vi "Field_C process Set field cmd.vi"(7 "Magnet Constants":T8, 10 "PSU Status in":T1 {"Trip Current" format="%.3f"; "Trip Field" format="%.4f"; "Voltage" format="%.2f"; "Field Constant" format="%.6f"; "MID Setpoint (T)" format="%.4f"; "MID Setpoint (A)" format="%.3f"; "MAX Setpoint (T)" format="%.4f"; "MAX Setpoint (A)" format="%.3f"; "Heater Voltage" format="%.2f"; "V Limit (V)" format="%.2f"; "Ramp Rate (A/s)" format="%.3f"; "Output (A)" format="%.3f"; "Output (T)" format="%.4f"; "Persistent Current" format="%.3f"; "Persistent Field" format="%.4f"}, 11 "Overall status in":T4) -> (2 "PSU Status Out out":T1 {"Trip Current" format="%.3f"; "Trip Field" format="%.4f"; "Voltage" format="%.2f"; "Field Constant" format="%.6f"; "MID Setpoint (T)" format="%.4f"; "MID Setpoint (A)" format="%.3f"; "MAX Setpoint (T)" format="%.4f"; "MAX Setpoint (A)" format="%.3f"; "Heater Voltage" format="%.2f"; "V Limit (V)" format="%.2f"; "Ramp Rate (A/s)" format="%.3f"; "Output (A)" format="%.3f"; "Output (T)" format="%.4f"; "Persistent Current" format="%.3f"; "Persistent Field" format="%.4f"}, 3 "Overall status out":T4)   [LabVIEW 2024, in "Magnet module.lvlib"]
uses:
  Magnet module.lvlib
  ctl/Magnet mode public.ctl
  ctl/SetField data.ctl
  ctl/Magnet config constants.ctl
  ctl/Magnet mode.ctl
  ctl/RampingOutput.ctl
  ctl/Actual magnet state.ctl
  ctl/Overall status.ctl
  <instrlib>/SMS drivers/Public/PSU Status.ctl
  <instrlib>/SMS drivers/Cryogenic Ltd SMSXXX.lvlib
panel:
  in  "Set Field":T2
  in  "error in (no error)":errorcluster
  out "Cmd response":string
  out "error out":errorcluster
  in  "Command name":string
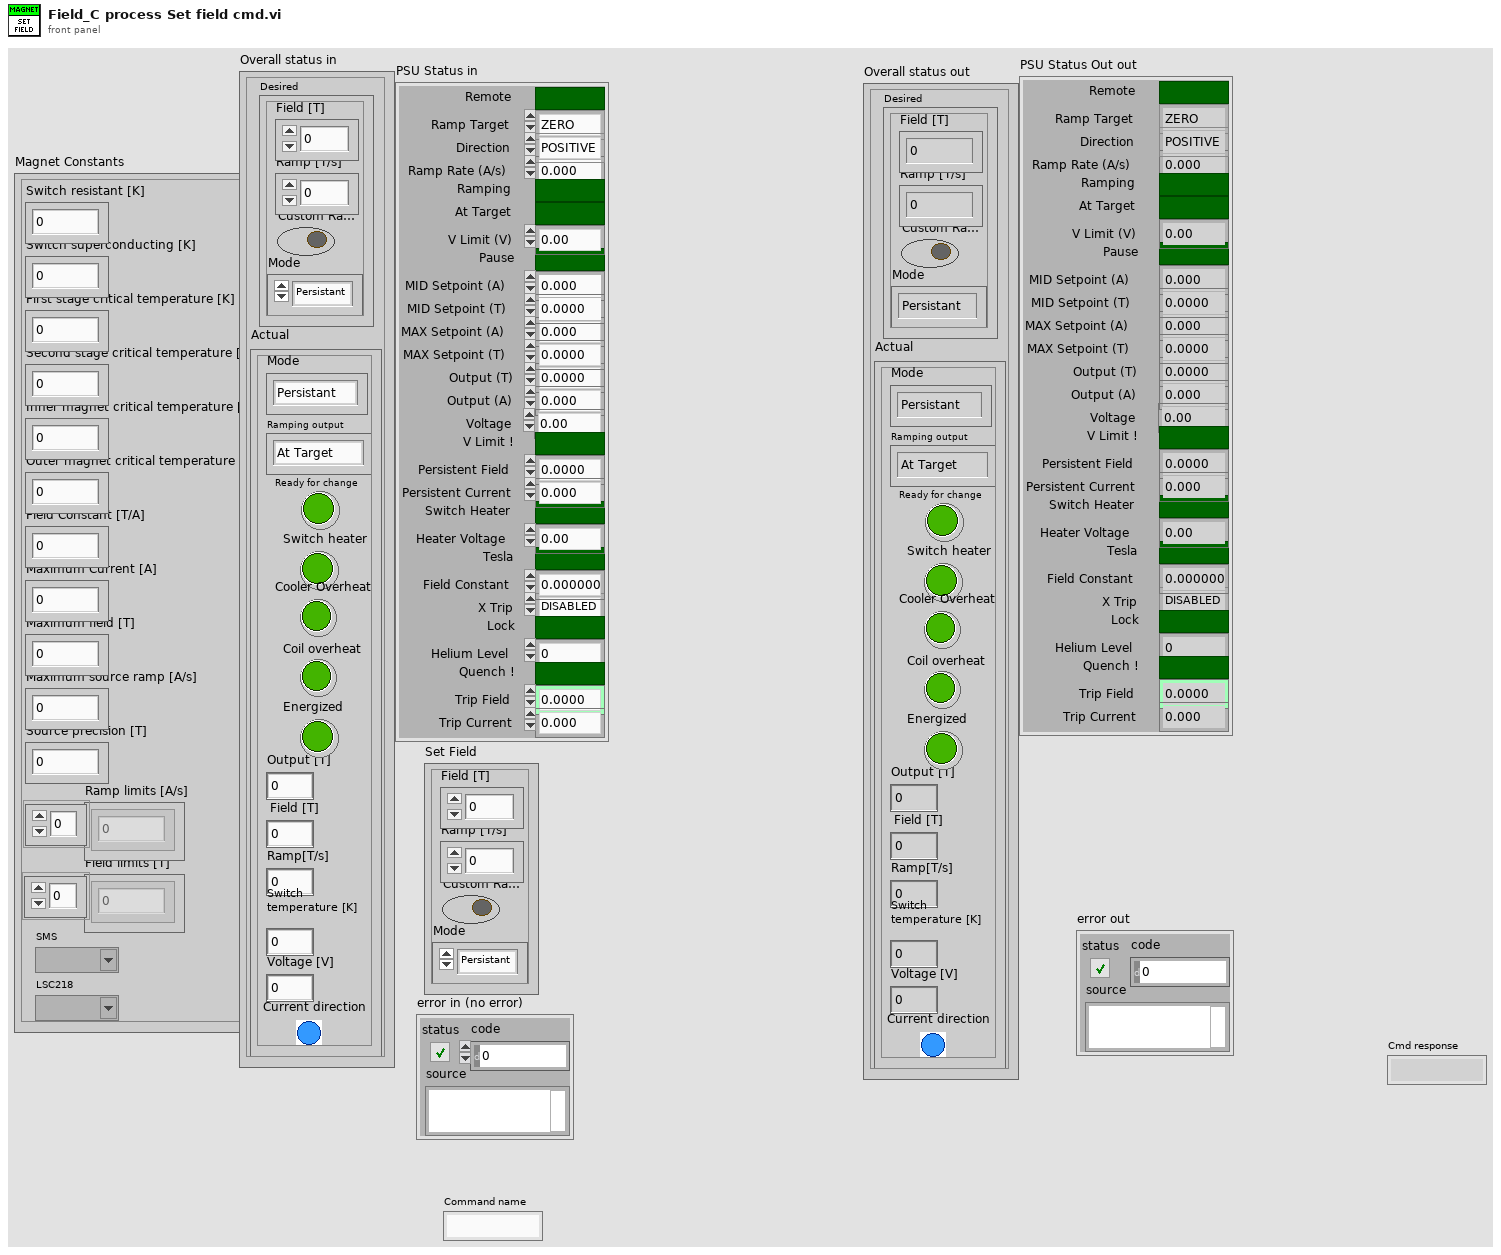
[diagram p1: front panel]
types:
  T1 = typedef "Cryogenic Ltd SMSXXX.lvlib/PSU Status.ctl" = cluster{"Ramp Target":enum16{"ZERO", "MID", "MAX"}, "Pause":bool, "Switch Heater":bool, "Persistent Field":dbl, "Persistent Current":dbl, "Tesla":bool, "Output (T)":dbl, "Output (A)":dbl, "X Trip":enum16{"DISABLED", "ENABLED", "ACTIVE"}, "Ramp Rate (A/s)":dbl, "V Limit (V)":dbl, "Heater Voltage":dbl, "MAX Setpoint (A)":dbl, "MAX Setpoint (T)":dbl, "MID Setpoint (A)":dbl, "MID Setpoint (T)":dbl, "Lock":bool, "Field Constant":dbl, "Remote":bool, "Direction":enum16{"POSITIVE", "NEGATIVE", "OPEN", "UNIPOLAR"}, "Helium Level":u16, "Quench !":bool, "Voltage":dbl, "V Limit !":bool, "Ramping":bool, "At Target":bool, "Trip Field":dbl, "Trip Current":dbl}
  T2 = typedef "Magnet module.lvlib/SetField data.ctl" = cluster{"Field [T]":dbl, "Ramp [T/s]":dbl, "Custom Ramp?":bool, "Mode":T3}
  T3 = typedef "Magnet module.lvlib/Magnet mode public.ctl" = enum16{"Persistant", "Ramping"}
  T4 = typedef "Magnet module.lvlib/Overall status.ctl" = cluster{"Desired":T2, "Actual":T5}
  T5 = typedef "Magnet module.lvlib/Actual magnet state.ctl" = cluster{"Mode":T6, "Ramping output":T7, "Ready for change":bool, "Switch heater":bool, "Cooler Overheat":bool, "Coil overheat":bool, "Energized":bool, "Output [T]":dbl, "Field [T]":dbl, "Ramp[T/s]":dbl, "Switch\ntemperature [K]":dbl, "Voltage [V]":dbl, "Current direction":bool}
  T6 = typedef "Magnet module.lvlib/Magnet mode.ctl" = enum16{"Persistant", "Switching", "Ramping", "Quenched"}
  T7 = typedef "Magnet module.lvlib/RampingOutput.ctl" = enum16{"At Target", "Go up", "Go down"}
  T8 = typedef "Magnet module.lvlib/Magnet config constants.ctl" = cluster{"Switch resistant [K]":dbl, "Switch superconducting [K]":dbl, "First stage critical temperature [K]":dbl, "Second stage critical temperature [K]":dbl, "Inner magnet critical temperature [K]":dbl, "Outer magnet critical temperature [K]":dbl, "Field Constant [T/A]":dbl, "Maximum Current [A]":dbl, "Maximum field [T]":dbl, "Maximum source ramp [A/s]":dbl, "Source precision [T]":dbl, "Ramp limits [A/s]":dbl[], "Field limits [T]":dbl[], "SMS":refnum<visa-resource-name>, "LSC218":refnum<visa-resource-name>}
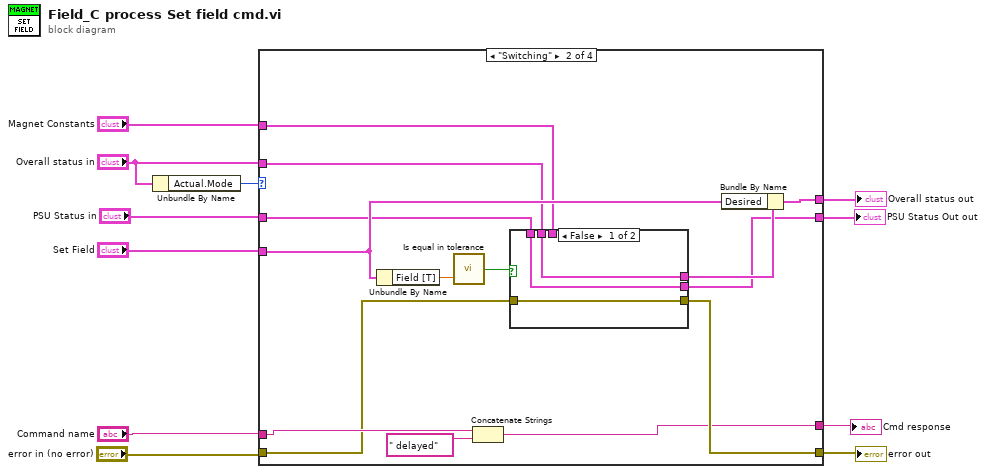
[diagram p0: block diagram]
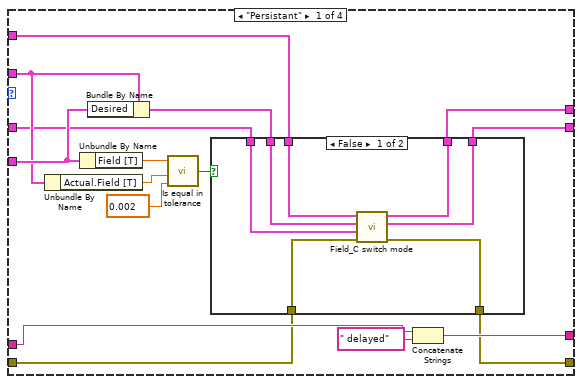
[diagram p2: hidden frame]
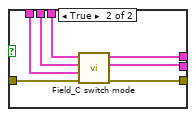
[diagram p4: hidden frame]
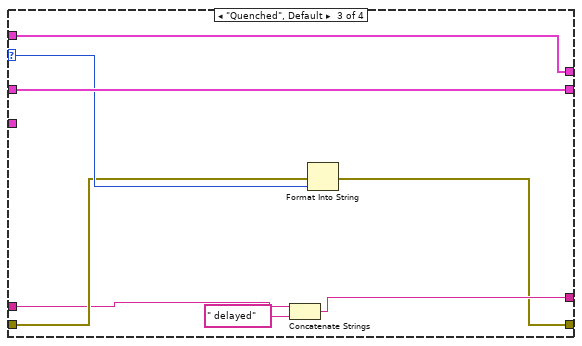
[diagram p5: hidden frame]
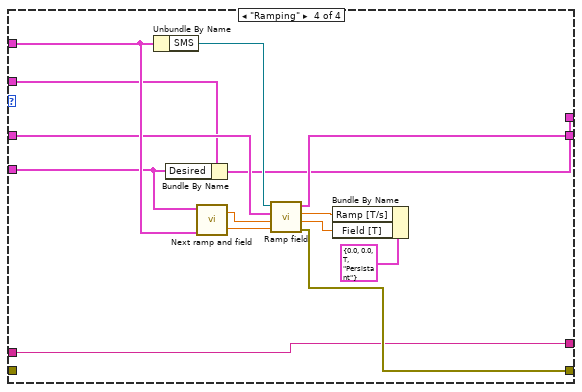
[diagram p6: hidden frame]
diagram:
  n1 = Unbundle By Name("Overall status in") -> ("Actual.Mode"=w1:T6)
  n2 = case shown="\"Switching\"" w1 {
    selector: w1 -> [_ _ w66 _]
    tunnel: "Overall status in" -> [w21 w47 w68 w73]
    tunnel: "Magnet Constants" -> [w18 w48 _ w83]
    tunnel: "PSU Status in" -> [w17 w46 w69 w82]
    tunnel: [w12 w43 w69 w81] -> w6
    tunnel: "Set Field" -> [w24 w49 _ w80]
    tunnel: "error in (no error)" -> [w16 w42 w65 _]
    tunnel: [w13 w51 w68 w71] -> w8
    tunnel: [w25 w39 w67 w70] -> w9
    tunnel: [w15 w41 w64 w72] -> w10
    tunnel: "Command name" -> [w26 w50 w63 w70]
    frame "Persistant" {
      n3 = Unbundle By Name(w21) -> ("Actual.Field [T]"=w20:dbl)
      n4 = Unbundle By Name(w24) -> ("Field [T]"=w23:dbl)
      n5 = Bundle By Name(cluster=w21, "Desired"=w24) -> (w14:T4)
      n6 = call "Is equal in tolerance.vi"("Absolut tolerance"=0.002, "Reference value"=w20, "Input value"=w23) -> ("Is in range"=w19:bool)  [unwired: 1 in]
      n7 = case shown="False" w19 {
        tunnel: w18 -> [w34 _]
        tunnel: w17 -> [w33 w36]
        tunnel: w16 -> [w32 w35]
        tunnel: [w31 w35] -> w15
        tunnel: w14 -> [w30 w37]
        tunnel: [w29 w37] -> w13
        tunnel: [w28 w36] -> w12
        frame False {
          n8 = call "Field_C switch mode.vi"("error in (no error)"=w32, "PSU Status"=w33, "Overall status in"=w30, "Magnet Constants"=w34) -> ("error out"=w31:errorcluster, "PSU Status out"=w28:T1, "Overall status out"=w29:T4)  [unwired: 5 in]
        }
        frame True {
        }
      }
      n9 = Concatenate Strings(w26, " delayed" ("string")) -> (w25:string)
    }
    frame "Switching" {
      n10 = Unbundle By Name(w49) -> ("Field [T]"=w45:dbl)
      n11 = call "Is equal in tolerance.vi"("Reference value"=w45) -> ("Is in range"=w40:bool)  [unwired: 3 in]
      n12 = Concatenate Strings(w50, " delayed" ("string")) -> (w39:string)
      n13 = case shown="False" w40 {
        tunnel: w48 -> [_ w61]
        tunnel: w47 -> [w53 w60]
        tunnel: w46 -> [w52 w59]
        tunnel: [w53 w58] -> w44
        tunnel: [w52 w57] -> w43
        tunnel: w42 -> [w54 w56]
        tunnel: [w54 w55] -> w41
        frame False {
        }
        frame True {
          n14 = call "Field_C switch mode.vi"("error in (no error)"=w56, "PSU Status"=w59, "Overall status in"=w60, "Magnet Constants"=w61) -> ("error out"=w55:errorcluster, "PSU Status out"=w57:T1, "Overall status out"=w58:T4)  [unwired: 5 in]
        }
      }
      n15 = Bundle By Name(cluster=w44, "Desired"=w49) -> (w51:T4)
    }
    frame "Quenched", Default {
      n16 = Concatenate Strings(w63, " delayed" ("string")) -> (w67:string)
      n17 = Format Into String(error in=w65, w66) -> (error out=w64:errorcluster)  [unwired: 2 in, 1 out]
    }
    frame "Ramping" {
      n18 = Unbundle By Name(w83) -> ("SMS"=w79:refnum<visa-resource-name>)
      n19 = Bundle By Name(cluster=w73, "Desired"=w80) -> (w71:T4)
      n20 = call "Next ramp and field.vi"("Magnet Constants in"=w83, "Desired"=w80) -> ("Ramp to set [A/s]"=w77:dbl, "Field to set [T]"=w78:dbl)  [unwired: 2 in]
      n21 = call "Ramp field.vi"("Ramp to set [A/s]"=w77, "Field to set [T]"=w78, "PSU Status In"=w82, "VISA Refnum in"=w79) -> ("error out"=w72:errorcluster, "Desired field (T)"=w75:dbl, "Ramp Rate (T/s)"=w76:dbl, "PSU Status Out"=w81:T1)  [unwired: 4 in]
      n22 = Bundle By Name(cluster=T2 {"Field [T]"=0.0, "Ramp [T/s]"=0.0, "Custom Ramp?"=TRUE, "Mode"=enum."Persistant"} ("Desired"), "Ramp [T/s]"=w76, "Field [T]"=w75) -> ()  [unwired: 1 out]
    }
  }
  "error out" <- w10
  "Cmd response" <- w9
  "Overall status out" <- w8
  "PSU Status Out out" <- w6
